vi "dsf components directory property name.vi"() -> (3 "components directory property name":string)   [LabVIEW 2019, in "DSF Shared.lvlib"]
uses:
  Shared/DSF Shared.lvlib
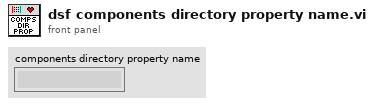
[diagram p1: front panel]
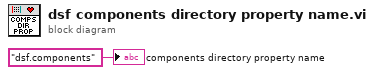
[diagram p0: block diagram]
diagram:
  "components directory property name" <- "dsf.components" ("Property Name")
